vi "FGV RTFIFO HW.vi"(8 "error in":errorcluster, 10 "Set?":bool, 11 "RT FIFO IN":refnum<k33>) -> (0 "error out":errorcluster, 3 "RT FIFO OUT":refnum<k33>)   [LabVIEW 2021, in "RT Main.lvlib"]
uses:
  RT Main.lvlib
  Libraries/Common RT/Hardware Monitoring.ctl
  Libraries/Common RT/Common RT.lvlib
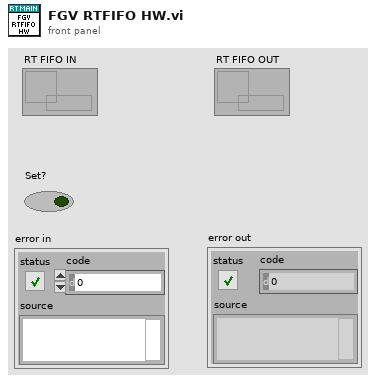
[diagram p1: front panel]
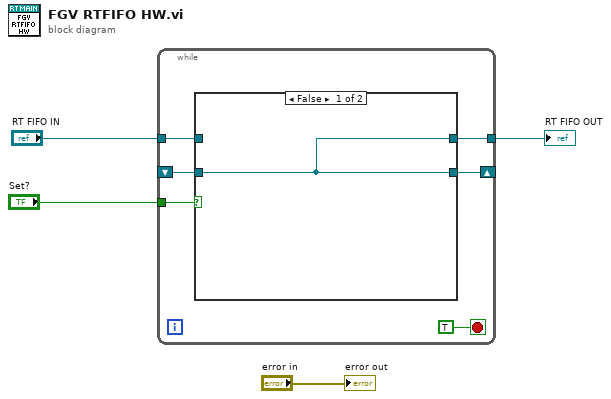
[diagram p0: block diagram]
diagram:
  n1 = while {
    tunnel: "Set?" -> [w9]
    tunnel: "RT FIFO IN" -> [w8]
    tunnel: [w7] -> w1
    shift-right: [w6] -> _
    shift-left: _ -> [w5]
    stop <- TRUE stop-if-true
    n2 = case shown="False" w9 {
      tunnel: w8 -> [_ w12]
      tunnel: [w11 w12] -> w7
      tunnel: [w11 w12] -> w6
      tunnel: w5 -> [w11 _]
      frame False {
      }
      frame True {
      }
    }
  }
  "RT FIFO OUT" <- w1
  "error out" <- "error in"
